vi "ReceiveStatusData.vi"(8 "error in":errorcluster, 10 "Timeout (ms)":i32, 11 "Connection In":T2={"UDP Connection ID"=refnum, "TCP Connection ID"=refnum, "Remote UDP Port"=61557, "Remote IP"=0}) -> (0 "error out":errorcluster, 2 "ClientStatusData":T1 {"gameState" items=["Start", "Pause", "Stop", "Close"]}, 3 "Connection Out":T2={"UDP Connection ID"=refnum, "TCP Connection ID"=refnum, "Remote UDP Port"=61557, "Remote IP"=0}, 4 "stop?":bool)   [LabVIEW 2017, in "Game.lvlib" / "GameComms.lvlib"]
uses:
  GameComms.lvlib
  TypeDefs/Connection.ctl
  TypeDefs/ClientStatusData.ctl
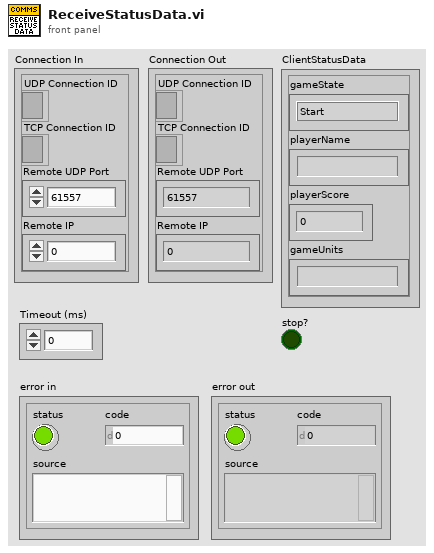
[diagram p1: front panel]
types:
  T1 = typedef "Game.lvlib/GameComms.lvlib/ClientStatusData.ctl" = cluster{"gameState":u16, "playerName":string, "playerScore":dbl, "gameUnits":string}
  T2 = typedef "Game.lvlib/GameComms.lvlib/Connection.ctl" = cluster{"UDP Connection ID":refnum<k16>, "TCP Connection ID":refnum<k5>, "Remote UDP Port":u16, "Remote IP":u32}
  T3 = enum16{"Standard", "Buffered", "CRLF", "Immediate"}
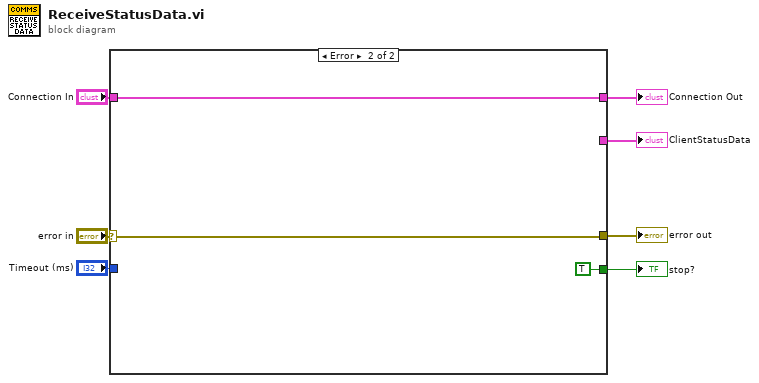
[diagram p0: block diagram]
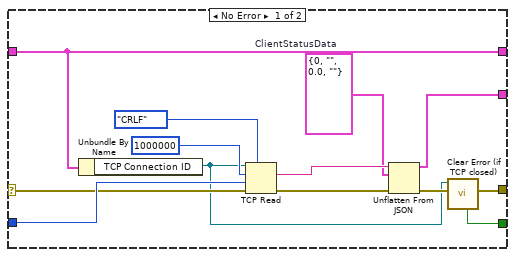
[diagram p2: hidden frame]
diagram:
  n1 = case shown="Error" "error in" {
    selector: "error in" -> [w18 w23]
    tunnel: [w9 w23] -> w6
    tunnel: "Connection In" -> [w17 w22]
    tunnel: [w17 w22] -> w4
    tunnel: "Timeout (ms)" -> [w19 _]
    tunnel: [w15 _] -> w2
    tunnel: [w8 TRUE ("stop?")] -> w1
    frame No Error {
      w16 = T1 {"gameState"=0, "playerName"="", "playerScore"=0.0, "gameUnits"=""}  # ClientStatusData
      n2 = Unbundle By Name(w17) -> ("TCP Connection ID"=w10:refnum<k5>)
      n3 = TCP Read(connection ID=w10, bytes to read=1000000, error in (no error)=w18, 7:T3."CRLF" ("mode (standard)"), 9:w19) -> (data out=w20:string, error out=w12:errorcluster)  [unwired: 1 out]
      n4 = Unflatten From JSON(JSON string=w20, type and defaults=w16, error in (no error)=w12) -> (value=w15:T1, error out=w11:errorcluster)  [unwired: 4 in]
      n5 = call "Clear Error (if TCP closed).vi"("error in"=w11, "tcp refnum"=w10) -> ("error out"=w9:errorcluster, "stop?"=w8:bool)  [unwired: 8 in]
    }
    frame Error {
    }
  }
  "error out" <- w6
  "Connection Out" <- w4
  "ClientStatusData" <- w2
  "stop?" <- w1
